vi "XW_Tutu_Chevray_PN.vi"() -> (5 "Plug in titles":string[](array[string]), 7 "Plug in values":string[](array[string]))   [LabVIEW 2010]
uses:
  Controls/Analysis_type_Enum.ctl
  Globals/Meas_global.vi
  <vilib>/Utility/file.llb/Read From Spreadsheet File (string).vi
panel:
  out "UW":bool
  out "Converged":bool=TRUE
  out "Third":dbl format="%#.3f"
  out "Filename":string
  out "Third Component":path
  out "Info index":i32
  out "2nd Comp":string
  out "1st Comp":string
  out "Psi 2":dbl=-999.0 format="%.2f"
  out "Psi 1":dbl=-999.0 format="%.2f"
  out "Indicies":i32[](array[numeric])
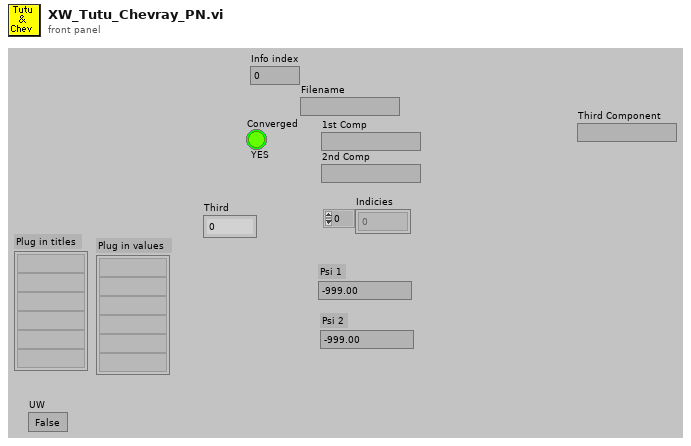
[diagram p1: front panel]
types:
  T1 = typedef "Correlation_cluster.ctl" = cluster{"U inst":string, "W inst":string, "uw":dbl, "uw/u'w'":dbl, "u^2w":dbl, "uw^2":dbl, "uw^3":dbl, "u^3w":dbl, "u^2w^2":dbl}
  T2 = typedef "Velocity_cluster.ctl" = cluster{"Name":string, "U":dbl, "u^2":dbl, "u^3/(u^2)^(1.5)":dbl, "u^4/(u^2)^2 -3":dbl, "% u'/U":dbl, "Mean % Err":dbl, "u^4":dbl}
  T3 = typedef "Analysis_type_cluster.ctl" = cluster{"Analysis type":T4, "Indicies":i32[], "Name":string, "Inst Array":T5, "Info index":i32}
  T4 = typedef "Analysis_type_Enum.ctl" = enum16{"Slow Response", "Fast Response", "Weighted Fast Response", "Fast FID", "Weighted Fast FID", "Cross Wire", "Weighted Cross Wire", "Weighted LDA"}
  T5 = typedef "Instrument_Array.ctl" = enum16{"PWA", "LDA", "Analogue"}
  T6 = enum16{"Save no data", "Save data in new files", "Save data in existing files"}
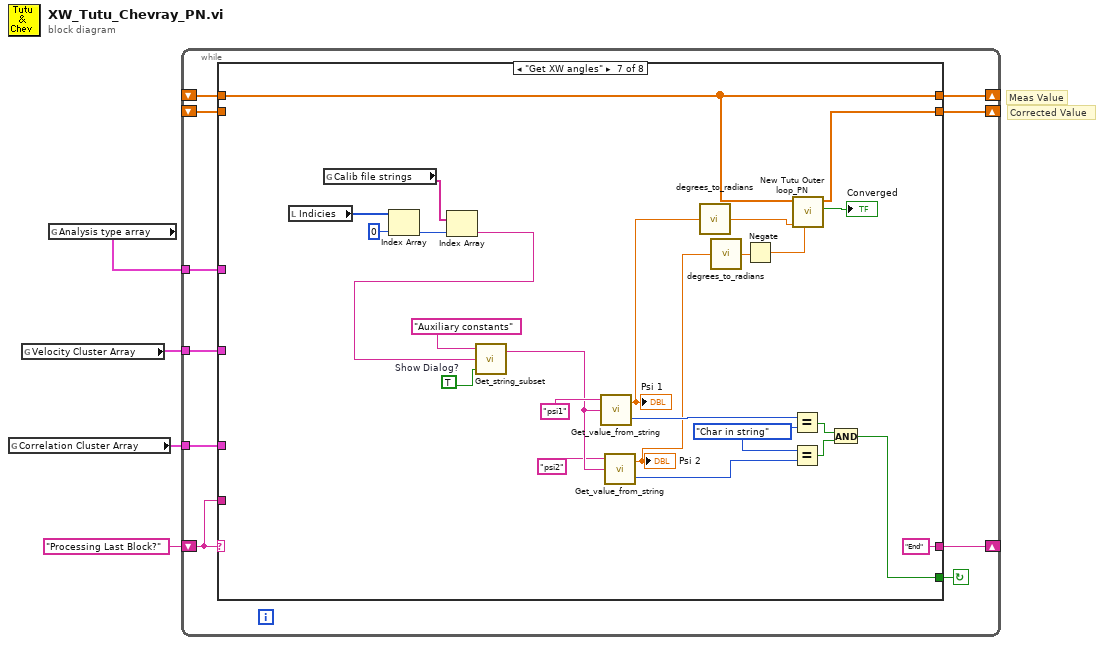
[diagram p0: block diagram]
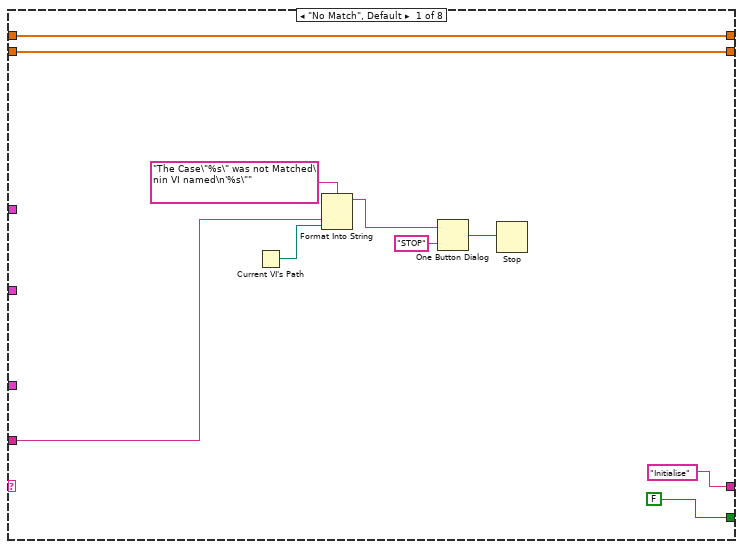
[diagram p2: hidden frame]
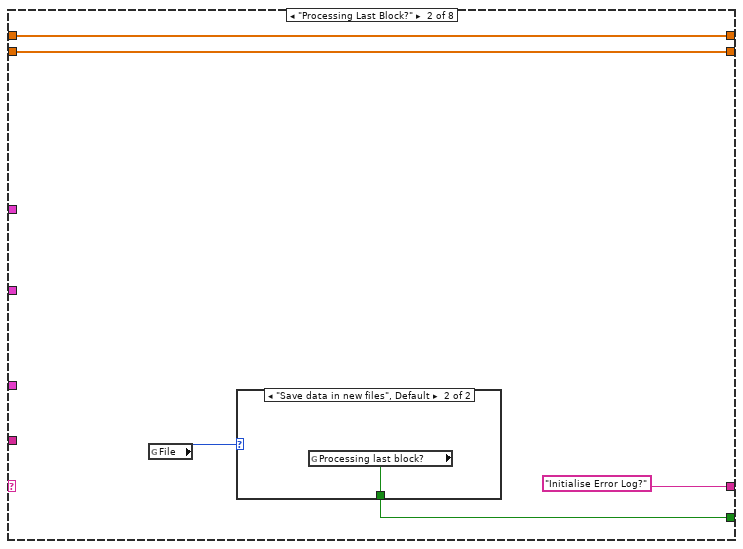
[diagram p3: hidden frame]
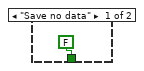
[diagram p4: hidden frame]
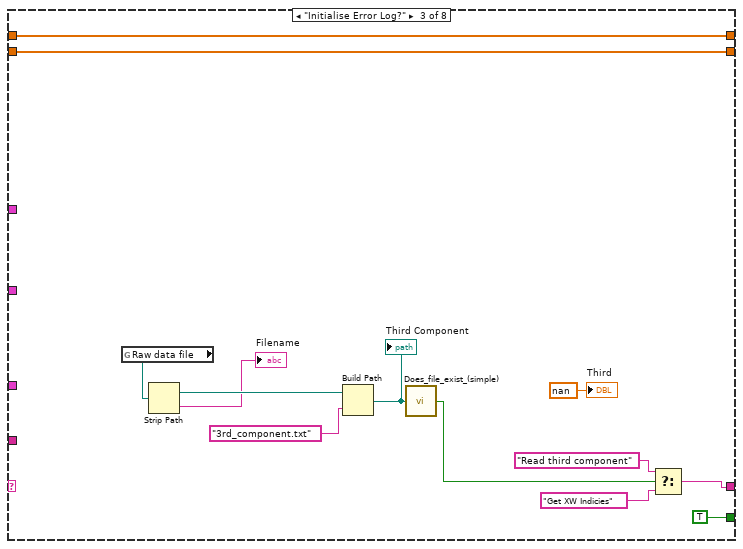
[diagram p5: hidden frame]
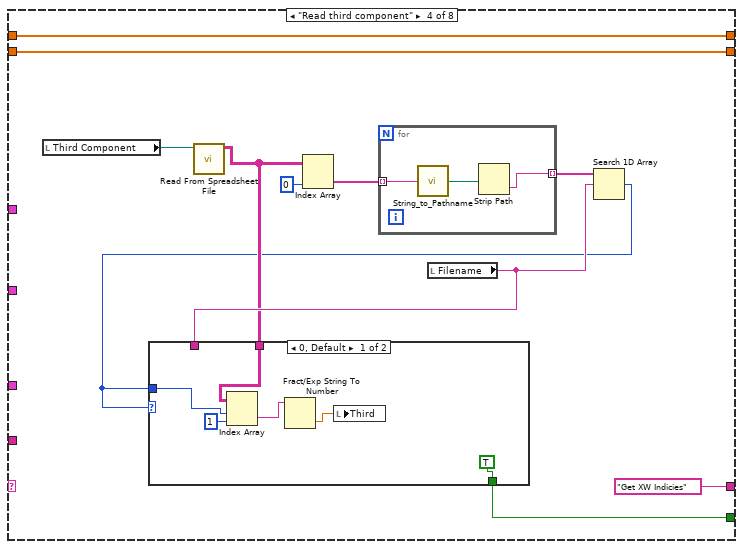
[diagram p6: hidden frame]
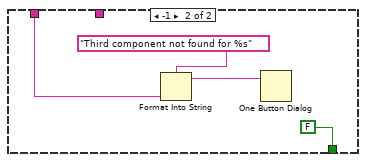
[diagram p7: hidden frame]
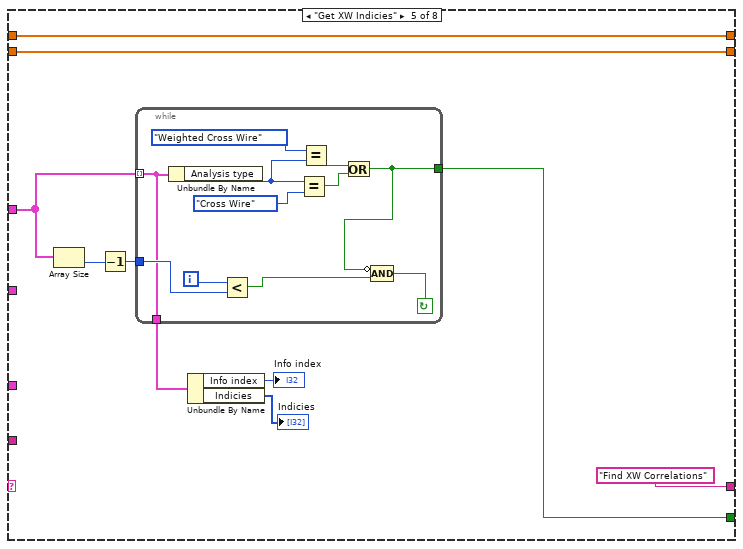
[diagram p8: hidden frame]
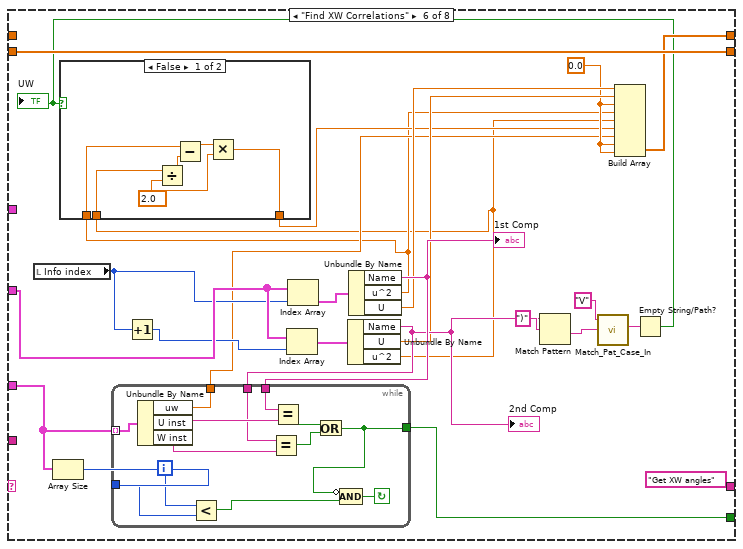
[diagram p9: hidden frame]
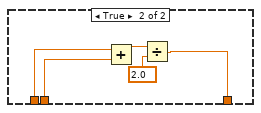
[diagram p10: hidden frame]
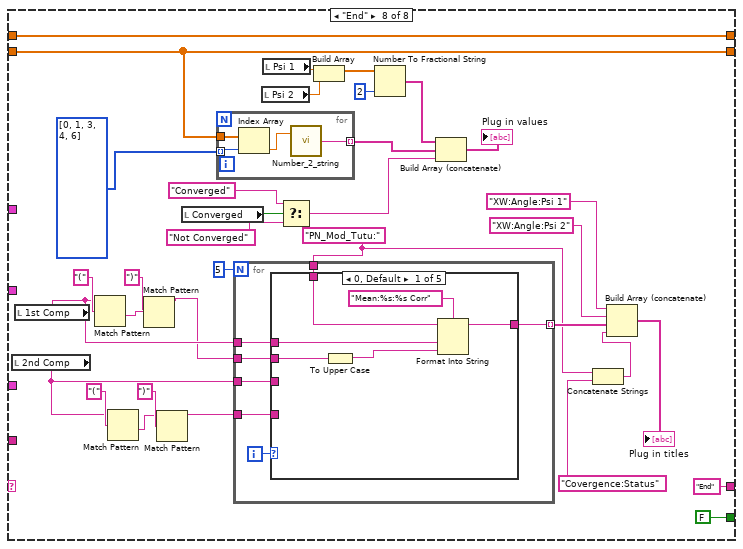
[diagram p11: hidden frame]
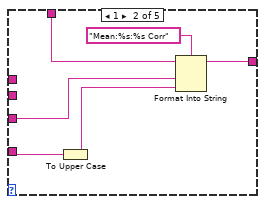
[diagram p12: hidden frame]
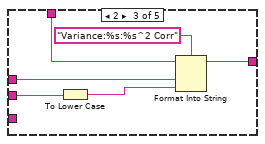
[diagram p13: hidden frame]
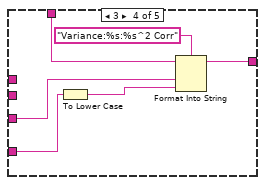
[diagram p14: hidden frame]
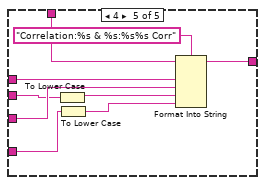
[diagram p15: hidden frame]
diagram:
  # "Corrected Value"
  # "Meas Value"
  n1 = global read "Meas_global.vi" "Correlation Cluster Array"() -> (w1:T1[])
  n2 = global read "Meas_global.vi" "Velocity Cluster Array"() -> (w2:T2[])
  n3 = global read "Meas_global.vi" "Analysis type array"() -> (w3:T3[])
  n4 = while {
    tunnel: w1 -> [w6]
    tunnel: w2 -> [w7]
    tunnel: w3 -> [w11]
    shift-left: _ -> [w5]
    shift-right: [w8] -> _
    shift-left: _ -> [w9]
    shift-right: [w10] -> _
    shift-left: "Processing Last Block?" -> [w12]
    shift-right: [w13] -> _
    stop <- w14 continue-if-true
    n5 = case shown="\"Get XW angles\"" w12 {
      tunnel: [FALSE w28 TRUE ("Processing last block?") w47 w73 w99 w147 FALSE ("Processing last block?")] -> w14
      tunnel: ["Initialise" "Initialise Error Log?" w34 "Get XW Indicies" "Find XW Correlations" "Get XW angles" "End" "End"] -> w13
      tunnel: w12 -> [w19 _ _ _ _ _ _ _]
      tunnel: w11 -> [_ _ _ _ w77 _ _ _]
      tunnel: [w16 w27 w44 w55 w72 w101 w146 w195] -> w10
      tunnel: w9 -> [w16 w27 w44 w55 w72 _ w146 w195]
      tunnel: [w15 w25 w43 w54 w71 w113 w145 w171] -> w8
      tunnel: w7 -> [_ _ _ _ _ w110 _ _]
      tunnel: w6 -> [_ _ _ _ _ w109 _ _]
      tunnel: w5 -> [w15 w25 w43 w54 w71 w113 _ w171]
      frame "No Match", Default {
        n6 = Current VI's Path() -> (path=w18:path)
        n7 = Format Into String(format string="The Case\"%s\" was not Matched\nin VI named\n'%s\"" ("Format String"), w19, w18) -> (resulting string=w22:string)  [unwired: 2 in, 1 out]
        n8 = One Button Dialog(message=w22, button name ("OK")="STOP") -> (true=w20:bool)
        n9 = Stop(stop? (T)=w20) -> ()
      }
      frame "Processing Last Block?" {
        n10 = global read "Meas_global.vi" "File"() -> (w26:T6)
        n11 = case shown="\"Save data in new files\", Default" w26 {
          tunnel: [FALSE ("Processing last block?") w31] -> w28
          frame "Save no data" {
          }
          frame "Save data in new files", Default {
            n12 = global read "Meas_global.vi" "Processing last block?"() -> (w31:bool)
          }
        }
      }
      frame "Initialise Error Log?" {
        n13 = global read "Meas_global.vi" "Raw data file"() -> (w41:path)
        n14 = Strip Path(path=w41) -> (stripped path=w40:path, name=→"Filename":string)
        n15 = Build Path(base path=w40, name or relative path="3rd_component.txt") -> (appended path=w38:path)
        "Third Component" <- w38
        n16 = call "Does_file_exist_(simple).vi"("Pathname"=w38) -> ("exists?"=w35:bool)
        n17 = Select(t="Read third component", s=w35, f="Get XW Indicies") -> (s? t:f=w34:string)
        "Third" <- nan ("Third")
      }
      frame "Read third component" {
        n18 = local read "Third Component"() -> (w52:path)
        n19 = call-poly <vilib>:"Read From Spreadsheet File.vi"("file path (dialog if empty)"=w52) -> ("all rows"=w46:string[][])  [unwired: 3 in, 7 out]
        n20 = Index Array(array=w46, index (col)=0 ("disabled index (col)")) -> (element=w50:string[])  [unwired: 1 in]
        n21 = for {
          tunnel: w50 -> [w68] mode=indexing
          tunnel: [w66] -> w49 mode=indexing
          n22 = call "String_to_Pathname.vi"("Input String"=w68) -> ("path"=w67:path)
          n23 = Strip Path(path=w67) -> (name=w66:string)  [unwired: 1 out]
        }
        n24 = local read "Filename"() -> (w48:string)
        n25 = Search 1D Array(1D array=w49, element=w48) -> (index of element=w45:i32)  [unwired: 1 out]
        n26 = case shown="0, Default" w45 {
          tunnel: w48 -> [_ w65]
          tunnel: [TRUE ("Processing last block?") FALSE ("Processing last block?")] -> w47
          tunnel: w46 -> [w59 _]
          tunnel: w45 -> [w58 _]
          frame 0, Default {
            n27 = Index Array(array=w59, index (row)=w58, index (col)=1 ("disabled index (col)")) -> (element=w57:string)
            n28 = Fract/Exp String To Number(string=w57) -> (number=w56:dbl)  [unwired: 4 out]
            n29 = local write "Third"(w56) -> ()
          }
          frame -1 {
            n30 = Format Into String(format string="Third component not found for %s" ("message"), w65) -> (resulting string=w63:string)  [unwired: 2 in, 1 out]
            n31 = One Button Dialog(message=w63) -> ()  [unwired: 2 out]
          }
        }
      }
      frame "Get XW Indicies" {
        n32 = Array Size(array=w77) -> (size(s)=w76:i32)
        n33 = Decrement(x=w76) -> (x-1=w75:i32)
        n34 = while {
          tunnel: [w79] -> w73
          tunnel: [w80] -> w74
          tunnel: w75 -> [w83]
          tunnel: w77 -> [w80] mode=indexing
          i -> [w84]
          stop <- w81 continue-if-true
          n35 = Unbundle By Name(w80) -> ("Analysis type"=w88:T4)
          n36 = Less?(x=w84, y=w83) -> (x < y?=w82:bool)
          n37 = Equal?(x=w88, y=Analysis_type_Enum."Cross Wire" ("Analysis type")) -> (x = y?=w86:bool)
          n38 = Equal?(x=Analysis_type_Enum."Weighted Cross Wire" ("Analysis type"), y=w88) -> (x = y?=w85:bool)
          n39 = Or(x=w85, y=w86) -> (x .or. y?=w79:bool)
          n40 = Compound Arithmetic op=AND(invert w79, w82) -> (w81:bool)
        }
        n41 = Unbundle By Name(w74) -> ("Info index"=→"Info index":i32, "Indicies"=→"Indicies":i32[])
      }
      frame "Find XW Correlations" {
        w95 = 0.0 ("element")
        n42 = local read "Info index"() -> (w98:i32)
        n43 = Array Size(array=w109) -> (size(s)=w107:i32)
        n44 = Increment(x=w98) -> (x+1=w97:i32)
        n45 = Index Array(array=w110, index=w97) -> (element=w111:T2)
        n46 = Index Array(array=w110, index=w98) -> (element=w112:T2)
        n47 = Unbundle By Name(w111) -> ("Name"=w105:string, "U"=w96:dbl, "u^2"=w91:dbl)
        "2nd Comp" <- w105
        n48 = Unbundle By Name(w112) -> ("Name"=w108:string, "u^2"=w92:dbl, "U"=w100:dbl)
        "1st Comp" <- w108
        n49 = while {
          tunnel: [w126] -> w94
          tunnel: w105 -> [w127]
          tunnel: w108 -> [w128]
          tunnel: w109 -> [w131] mode=indexing
          tunnel: [w132] -> w99
          tunnel: w107 -> [w135]
          i -> [w136]
          stop <- w133 continue-if-true
          n50 = Unbundle By Name(w131) -> ("uw"=w126:dbl, "U inst"=w130:string, "W inst"=w129:string)
          n51 = Less?(x=w136, y=w135) -> (x < y?=w134:bool)
          n52 = Equal?(x=w127, y=w129) -> (x = y?=w138:bool)
          n53 = Equal?(x=w128, y=w130) -> (x = y?=w137:bool)
          n54 = Or(x=w137, y=w138) -> (x .or. y?=w132:bool)
          n55 = Compound Arithmetic op=AND(invert w132, w134) -> (w133:bool)
        }
        n56 = Match Pattern(string=w105, regular expression=")") -> (after substring=w103:string)  [unwired: 4 out]
        n57 = call "Match_Pat_Case_In.vi"("String to match"="V" ("regular expression"), "String"=w103) -> ("Matched string"=w102:string)  [unwired: 1 in, 3 out]
        n58 = Empty String/Path?(string/path=w102) -> (empty?=w90:bool)
        "UW" <- w90
        n59 = case shown="False" w90 {
          tunnel: w92 -> [w116 w122]
          tunnel: w91 -> [w115 w121]
          tunnel: [w117 w123] -> w93
          frame False {
            w118 = 2.0 ("y")
            n60 = Divide(x=w115, y=w118) -> (x/y=w120:dbl)
            n61 = Subtract(x=w116, y=w120) -> (x-y=w119:dbl)
            n62 = Multiply(x=w119, y=w118) -> (x*y=w117:dbl)
          }
          frame True {
            n63 = Add(x=w122, y=w121) -> (x+y=w125:dbl)
            n64 = Divide(x=w125, y=2.0) -> (x/y=w123:dbl)
          }
        }
        n65 = Build Array(w100, w96, w95, w92, w91, w93, w94, w95, w95) -> (w101:dbl[])
      }
      frame "Get XW angles" {
        w152 = enum16{"Char in string", "Char not in string"}."Char in string" ("Status")
        w158 = TRUE  # Show Dialog?
        n66 = local read "Indicies"() -> (w162:i32[])
        n67 = global read "Meas_global.vi" "Calib file strings"() -> (w161:string[])
        n68 = Index Array(array=w162, index=0 ("Index")) -> (element=w160:i32)
        n69 = Index Array(array=w161, index=w160) -> (element=w157:string)
        n70 = call "Get_string_subset.vi"("Show Dialog?"=w158, "String to split"=w157, "File Label"="Auxiliary constants") -> ("Output string"=w155:string)  [unwired: 1 in, 1 out]
        n71 = call "Get_value_from_string.vi"("Input string"=w155, "Variable name"="psi1") -> ("Status"=w151:enum16{"Char in string", "Char not in string"}, "Value"=w139:dbl)  [unwired: 1 in]
        "Psi 1" <- w139
        n72 = call "Get_value_from_string.vi"("Input string"=w155, "Variable name"="psi2") -> ("Status"=w150:enum16{"Char in string", "Char not in string"}, "Value"=w143:dbl)  [unwired: 1 in]
        "Psi 2" <- w143
        n73 = call "degrees_to_radians.vi"("degrees"=w139) -> ("radians"=w140:dbl)
        n74 = call "degrees_to_radians.vi"("degrees"=w143) -> ("radians"=w142:dbl)
        n75 = Negate(x=w142) -> (-x=w141:dbl)
        n76 = Equal?(x=w151, y=w152) -> (x = y?=w148:bool)
        n77 = Equal?(x=w152, y=w150) -> (x = y?=w149:bool)
        n78 = call "New Tutu Outer loop_PN.vi"("Const psi2"=w141, "Const psi1"=w140, "Measured stats"=w146) -> ("Converged"=→"Converged":bool, "Corrected stats"=w145:dbl[])  [unwired: 7 out]
        n79 = And(x=w148, y=w149) -> (x .and. y?=w147:bool)
      }
      frame "End" {
        w165 = "PN_Mod_Tutu:"
        n80 = local read "2nd Comp"() -> (w184:string)
        n81 = local read "1st Comp"() -> (w188:string)
        n82 = Match Pattern(string=w188, regular expression="(") -> (after substring=w193:string)  [unwired: 4 out]
        n83 = Match Pattern(string=w184, regular expression="(") -> (after substring=w189:string)  [unwired: 4 out]
        n84 = Match Pattern(string=w193, regular expression=")") -> (before substring=w187:string)  [unwired: 4 out]
        n85 = Match Pattern(string=w189, regular expression=")") -> (before substring=w183:string)  [unwired: 4 out]
        n86 = local read "Converged"() -> (w170:bool)
        n87 = for {
          tunnel: [w201] -> w173 mode=indexing
          tunnel: i32[] [0, 1, 3, 4, 6] -> [w200] mode=indexing
          tunnel: w171 -> [w198]
          n88 = Index Array(array=w198, index=w200) -> (element=w199:dbl)
          n89 = call "Number_2_string.vi"("number"=w199) -> ("String"=w201:string)  [unwired: 1 in]
        }
        n90 = for {
          N: 5 -> [_]
          tunnel: w165 -> [w207]
          tunnel: w188 -> [w206]
          tunnel: w187 -> [w205]
          tunnel: [w204] -> w186 mode=indexing
          tunnel: w184 -> [w203]
          tunnel: w183 -> [w202]
          i -> [w208]
          n91 = case shown="0, Default" w208 {
            tunnel: w207 -> [w209 w217 w221 w227 w233]
            tunnel: w206 -> [w211 _ w225 _ w238]
            tunnel: w205 -> [w213 _ w223 _ w236]
            tunnel: [w210 w218 w224 w231 w240] -> w204
            tunnel: w203 -> [_ w215 _ w229 w237]
            tunnel: w202 -> [_ w216 _ w228 w239]
            frame 0, Default {
              n92 = To Upper Case(1:w213) -> (0:w214:string)
              n93 = Format Into String(format string="Mean:%s:%s Corr" ("Format String"), initial string=w209, w211, w214) -> (resulting string=w210:string)  [unwired: 1 in, 1 out]
            }
            frame 1 {
              n94 = To Upper Case(1:w216) -> (0:w220:string)
              n95 = Format Into String(format string="Mean:%s:%s Corr" ("Format String"), initial string=w217, w215, w220) -> (resulting string=w218:string)  [unwired: 1 in, 1 out]
            }
            frame 2 {
              n96 = To Lower Case(string=w223) -> (all lower case string=w222:string)
              n97 = Format Into String(format string="Variance:%s:%s^2 Corr" ("Format String"), initial string=w221, w225, w222) -> (resulting string=w224:string)  [unwired: 1 in, 1 out]
            }
            frame 3 {
              n98 = To Lower Case(string=w228) -> (all lower case string=w230:string)
              n99 = Format Into String(format string="Variance:%s:%s^2 Corr" ("Format String"), initial string=w227, w229, w230) -> (resulting string=w231:string)  [unwired: 1 in, 1 out]
            }
            frame 4 {
              n100 = To Lower Case(string=w236) -> (all lower case string=w235:string)
              n101 = To Lower Case(string=w239) -> (all lower case string=w234:string)
              n102 = Format Into String(format string="Correlation:%s & %s:%s%s Corr" ("Format String"), initial string=w233, w238, w237, w235, w234) -> (resulting string=w240:string)  [unwired: 1 in, 1 out]
            }
          }
        }
        n103 = local read "Psi 2"() -> (w176:dbl)
        n104 = local read "Psi 1"() -> (w177:dbl)
        n105 = Select(t="Converged", s=w170, f="Not Converged") -> (s? t:f=w167:string)
        n106 = Build Array(w177, w176) -> (w175:dbl[])
        n107 = Number To Fractional String(number=w175, precision (6)=i16 2) -> (F-format string=w174:string[])  [unwired: 2 out]
        n108 = Build Array (concatenate)(w174, w173, w167) -> (→"Plug in values":string[])
        n109 = Concatenate Strings(w165, "Covergence:Status" ("string")) -> (w166:string)
        n110 = Build Array (concatenate)("XW:Angle:Psi 1", "XW:Angle:Psi 2", w186, w166) -> (→"Plug in titles":string[])
      }
    }
  }
